vi "variable_length_value.vi"(11 "datastream in":u8[](array[numeric]) format="%08x") -> (2 "Variable Length Value":u32, 3 "datastream out":u8[](array[numeric]) format="%.0x")   [LabVIEW 2020, in "midi-file.lvclass"]
uses:
  midi-file.lvclass
  midi-file.lvclass/midi-file.ctl
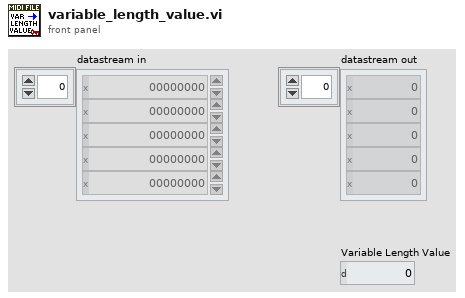
[diagram p1: front panel]
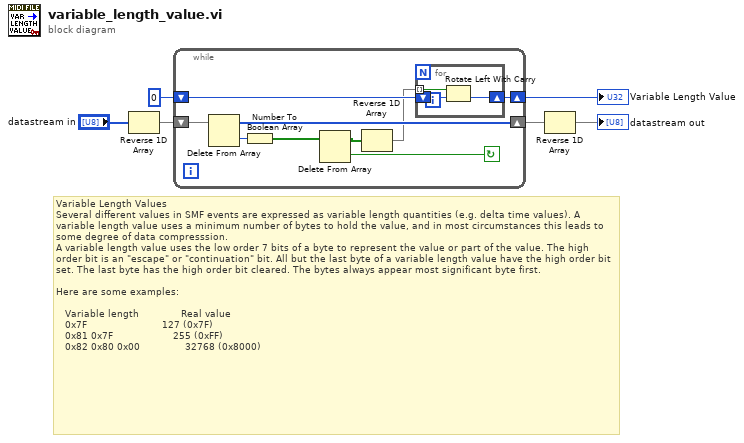
[diagram p0: block diagram]
diagram:
  # "Variable Length Values\nSeveral different values in SMF events are expressed as variable length quantities (e.g. delta time values). A variable length value uses a minimum number of bytes to hold the value, and in most circumstances this leads to some degree of data compresssion.\nA variable length value uses the low order 7 bits of a byte to represent the value or part of the value. The high order bit is an \"escape\" or \"continuation\" bit. All but the last byte of a variable length value have the high order bit set. The last byte has the high order bit cleared. The bytes always appear most significant byte first.\n\nHere are some examples:\n\n   Variable length              Real value\n   0x7F                         127 (0x7F)\n   0x81 0x7F                    255 (0xFF)\n   0x82 0x80 0x00               32768 (0x8000)"
  n1 = Reverse 1D Array(array="datastream in") -> (reversed array=w4:u8[])
  n2 = while {
    shift-right: [w10] -> w1
    shift-left: u32 0 -> [w11]
    shift-right: [w12] -> w3
    shift-left: w4 -> [w14]
    stop <- w15 continue-if-true
    n3 = Delete From Array(array=w14) -> (deleted portion=w13:u8, array with subset deleted=w12:u8[])  [unwired: 2 in]
    n4 = Number To Boolean Array(number=w13) -> (Boolean array=w8:bool[])
    n5 = Delete From Array(array=w8) -> (deleted portion=w15:bool, array with subset deleted=w9:bool[])  [unwired: 2 in]
    n6 = Reverse 1D Array(array=w9) -> (reversed array=w7:bool[])
    n7 = for {
      tunnel: w7 -> [w17] mode=indexing
      shift-right: [w16] -> w10
      shift-left: w11 -> [w18]
      n8 = Rotate Left With Carry(2:w18, 3:w17) -> (0:w16:u32)  [unwired: 1 out]
    }
  }
  "Variable Length Value" <- w1
  n9 = Reverse 1D Array(array=w3) -> (reversed array=→"datastream out":u8[])
